vi "get ids from tree.vi"(8 "error in":errorcluster, 11 "Tree":string) -> (0 "error out":errorcluster, 3 "tags":variant)   [LabVIEW 2013, in "TreeRepresentation.lvlib"]
doc: "Tags der Baumstruktur auslesen"
uses:
  TreeRepresentation.lvlib
  <vilib>/regexp/Match Regular Expression.xnode
panel:
  in  "tags":variant
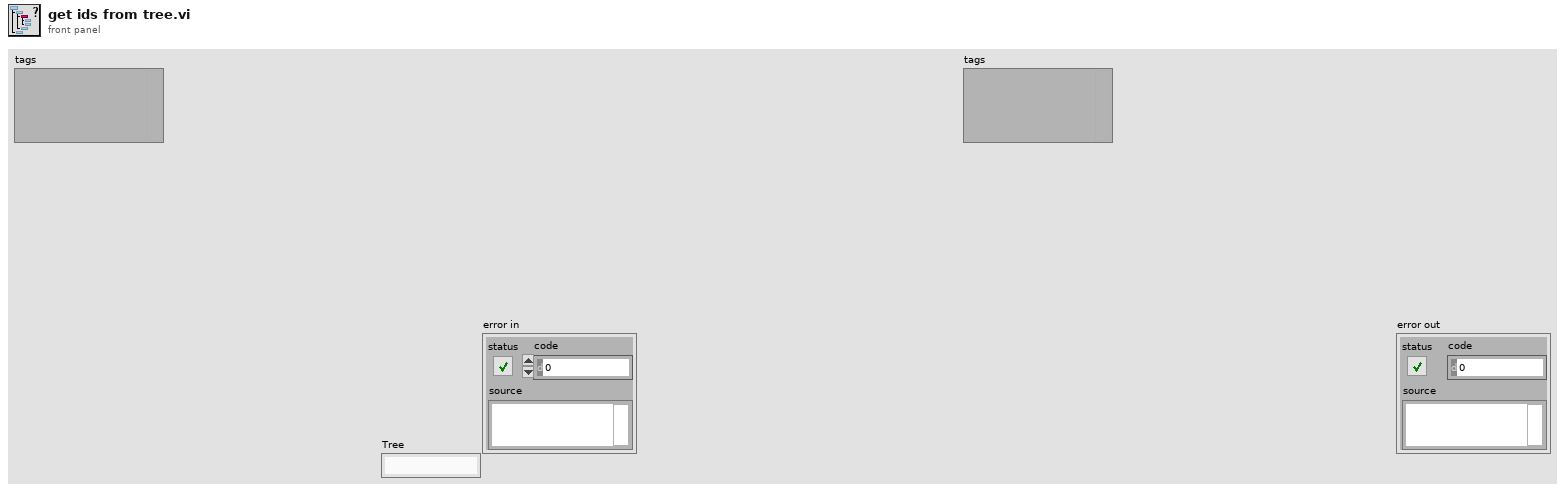
[diagram p1: front panel]
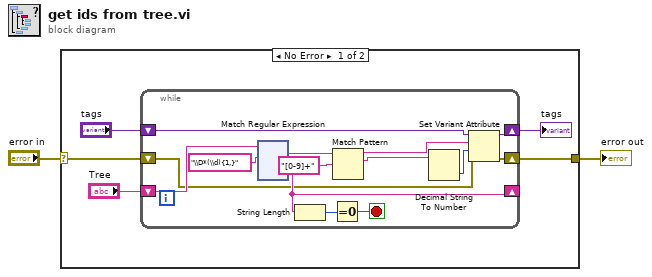
[diagram p0: block diagram]
diagram:
  n1 = case shown="No Error" "error in" {
    selector: "error in" -> [w4 w136]
    tunnel: [w3 w136] -> w1
    frame No Error {
      n2 = while {
        shift-right: [w19] -> _
        shift-left: "Tree" -> [w20]
        shift-right: [w10] -> w5
        shift-left: "tags" -> [w16]
        shift-right: [w8] -> w3
        shift-left: w4 -> [w9]
        stop <- w17 stop-if-true
        n3 = xnode "Match Regular Expression"("input string"=w20, "regular expression"="\\D*(\\d){1,}") -> ("whole match"=w15:string, "after match"=w19:string)  [unwired: 4 in, 3 out]
        n4 = String Length(string=w19) -> (length=w18:i32)
        n5 = Equal To 0?(x=w18) -> (x = 0?=w17:bool)
        n6 = Match Pattern(string=w15, regular expression="[0-9]+") -> (before substring=w13:string, match substring=w12:string)  [unwired: 1 in, 2 out]
        n7 = Decimal String To Number(string=w12) -> (number=w11:i32)  [unwired: 2 in, 1 out]
        n8 = Set Variant Attribute(Variant=w16, name=w13, value=w11, error in=w9) -> (Variant out=w10:variant, error out=w8:errorcluster)  [unwired: 1 out]
      }
      "tags" <- w5
    }
    frame Error {
    }
  }
  "error out" <- w1
